vi "subcollect.vi"(2 "Firing Data":T1={"error"={"status"=FALSE, "code"=0, "source"=""}, "LeftWheelRefnum"={"DeviceStatus"={"status"=FALSE, "code"=0, "source"=""}, "Type"=enum."PWM", "PWM"={"PWM Channel"=enum."Invalid", "DeadBand"={"Name"="", "maxPositivePwm"=0, "minPositivePwm"=0, "centerPwm"=0, "maxNegativePwm"=0, "minNegativePwm"=0, "angularRange"=0}}, "CAN"={"Device Number"=0, "Control Mode"=enum."Percent VBus", "Semaphore"=refnum, "Max Vout"=12.0, "TalonSRX Control Mode"=enum."Percent VBus"}, "Invert"=FALSE}, "RightWheelRefnum"={"DeviceStatus"={"status"=FALSE, "code"=0, "source"=""}, "Type"=enum."PWM", "PWM"={"PWM Channel"=enum."Invalid", "DeadBand"={"Name"="", "maxPositivePwm"=0, "minPositivePwm"=0, "centerPwm"=0, "maxNegativePwm"=0, "minNegativePwm"=0, "angularRange"=0}}, "CAN"={"Device Number"=0, "Control Mode"=enum."Percent VBus", "Semaphore"=refnum, "Max Vout"=12.0, "TalonSRX Control Mode"=enum."Percent VBus"}, "Invert"=FALSE}, "PushSolenoidRefnum"={"DevStatus"={"status"=FALSE, "code"=0, "source"=""}, "Pneumatics Control Module"=0, "Forward Solenoid Channel"=enum."Invalid", "Reverse Solenoid Channel"=enum."Invalid"}, "AngleMotorPosition(t)"=0.0, "LaunchSpeed(t/100ms)"=0.0, "CollectSpeed(t/100ms)"=0.0, "SpinupDuration(10ms)"=0, "ShotDuration(10ms)"=0, "PowerScale"=0.0, "AngleShift"=0, "VisionPrepAngle"=0.0}, 3 "Manual Control":T11, 4 "CollectionTrigger":bool, 5 "SpinupTrigger":bool) -> (0 "Speed":dbl, 1 "Angle":dbl)   [LabVIEW 2015]
uses:
  Bundle.ctl
  <vilib>/Rock Robotics/WPI/MotorControl/WPI_MotorControlDeviceRef.ctl
  <vilib>/Rock Robotics/WPI/MotorControl/WPI_MotorControlType.ctl
  <vilib>/Rock Robotics/SystemInterfaces/DIO/FPGA_DIOPWMChannel.ctl
  <vilib>/Rock Robotics/WPI/PWM/WPI_PWMDeadband.ctl
  <vilib>/Rock Robotics/WPI/CAN/Jaguar/SubVIs/WPI_CANJaguar_ControlMode.ctl
  <vilib>/Rock Robotics/WPI/CAN/TalonSRX/WPI_CANTalonSRX_APIControlMode.ctl
  <vilib>/Rock Robotics/WPI/Solenoid/WPI_SolenoidDevRef.ctl
  <vilib>/Rock Robotics/WPI/Solenoid/WPI_SolenoidChannel.ctl
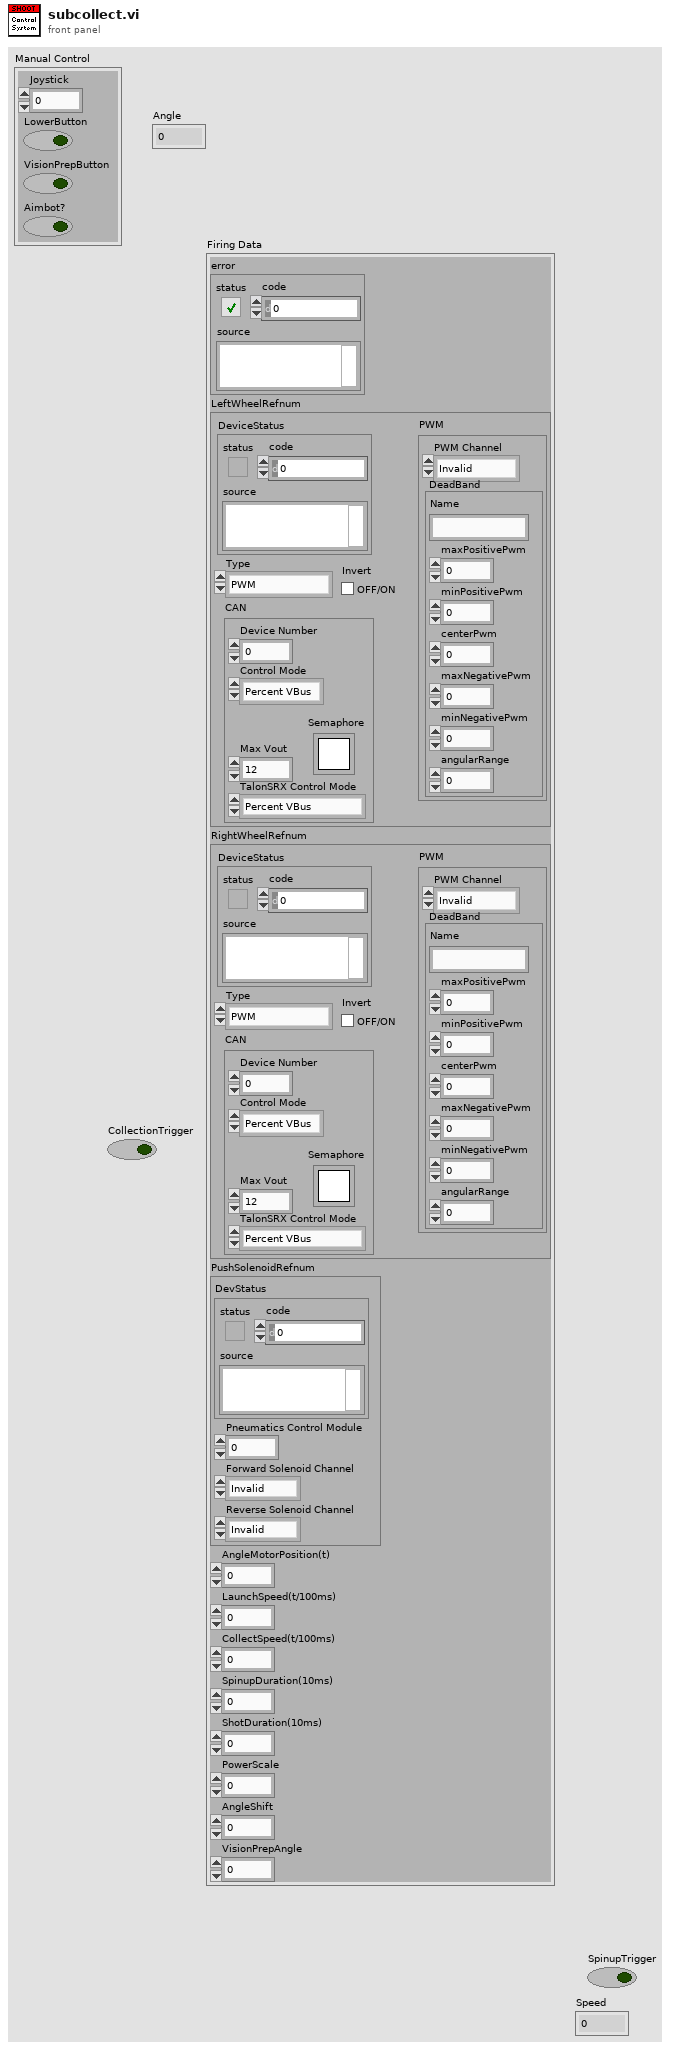
[diagram p1: front panel]
types:
  T1 = typedef "Bundle.ctl" = cluster{"error":errorcluster, "LeftWheelRefnum":T2, "RightWheelRefnum":T2, "PushSolenoidRefnum":T9, "AngleMotorPosition(t)":dbl, "LaunchSpeed(t/100ms)":dbl, "CollectSpeed(t/100ms)":dbl, "SpinupDuration(10ms)":i32, "ShotDuration(10ms)":i32, "PowerScale":dbl, "AngleShift":i32, "VisionPrepAngle":dbl}
  T2 = typedef "WPI_MotorControlDeviceRef.ctl" = cluster{"DeviceStatus":errorcluster, "Type":T3, "PWM":cluster{"PWM Channel":T4, "DeadBand":T5}, "CAN":cluster{"Device Number":u8, "Control Mode":T6, "Semaphore":T7, "Max Vout":dbl, "TalonSRX Control Mode":T8}, "Invert":bool}
  T3 = typedef "WPI_MotorControlType.ctl" = enum16{"PWM", "CAN", "CANTalonSRX"}
  T4 = typedef "FPGA_DIOPWMChannel.ctl" = enum8{"PWM 0", "PWM 1", "PWM 2", "PWM 3", "PWM 4", "PWM 5", "PWM 6", "PWM 7", "PWM 8", "PWM 9", "PWM MXP 0", "PWM MXP 1", "PWM MXP 2", "PWM MXP 3", "PWM MXP 4", "PWM MXP 5", "PWM MXP 6", "PWM MXP 7", "PWM MXP 8", "PWM MXP 9", "Invalid"}
  T5 = typedef "WPI_PWMDeadband.ctl" = cluster{"Name":string, "maxPositivePwm":i32, "minPositivePwm":i32, "centerPwm":i32, "maxNegativePwm":i32, "minNegativePwm":i32, "angularRange":u16}
  T6 = typedef "WPI_CANJaguar_ControlMode.ctl" = enum8{"Percent VBus", "Current", "Speed", "Position", "Voltage"}
  T7 = typedef "Semaphore RefNum" = refnum<k1>
  T8 = typedef "WPI_CANTalonSRX_APIControlMode.ctl" = enum8{"Percent VBus", "Speed", "Position", "Slave", "Unchanged / Invalid", "Voltage Compensation", "Current", "Motion Profile"}
  T9 = typedef "WPI_SolenoidDevRef.ctl" = cluster{"DevStatus":errorcluster, "Pneumatics Control Module":u8, "Forward Solenoid Channel":T10, "Reverse Solenoid Channel":T10}
  T10 = typedef "WPI_SolenoidChannel.ctl" = enum8{"Solenoid 0", "Solenoid 1", "Solenoid 2", "Solenoid 3", "Solenoid 4", "Solenoid 5", "Solenoid 6", "Solenoid 7", "Invalid"}
  T11 = cluster{"Joystick":dbl, "LowerButton":bool, "VisionPrepButton":bool, "Aimbot?":bool}
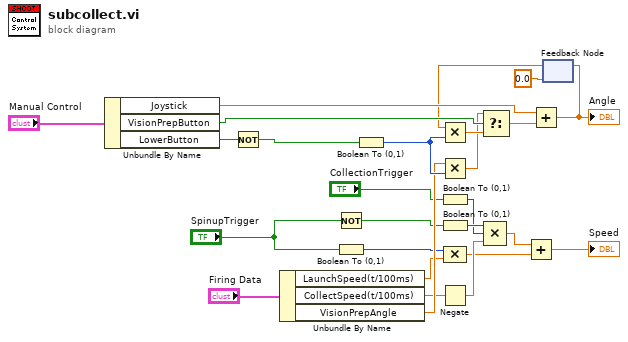
[diagram p0: block diagram]
diagram:
  n1 = Unbundle By Name("Manual Control") -> ("Joystick"=w19:dbl, "VisionPrepButton"=w26:bool, "LowerButton"=w25:bool)
  n2 = Not(x=w25) -> (.not. x?=w20:bool)
  n3 = Unbundle By Name("Firing Data") -> ("LaunchSpeed(t/100ms)"=w8:dbl, "CollectSpeed(t/100ms)"=w10:dbl, "VisionPrepAngle"=w16:dbl)
  n4 = Not(x="SpinupTrigger") -> (.not. x?=w11:bool)
  n5 = Boolean To (0,1)(Boolean="SpinupTrigger") -> (0, 1=w9:i16)
  n6 = Boolean To (0,1)(Boolean=w20) -> (0, 1=w22:i16)
  n7 = Multiply(x=w16, y=w22) -> (x*y=w21:dbl)
  n8 = Boolean To (0,1)(Boolean="CollectionTrigger") -> (0, 1=w14:i16)
  n9 = Boolean To (0,1)(Boolean=w11) -> (0, 1=w15:i16)
  n10 = Negate(x=w10) -> (-x=w13:dbl)
  n11 = Compound Arithmetic op=MULTIPLY(w9, w8) -> (w6:dbl)
  n12 = Compound Arithmetic op=MULTIPLY(w15, w14, w13) -> (w5:dbl)
  n13 = Add(x=w5, y=w6) -> (x+y=→"Speed":dbl)
  n14 = feedback #1(0.0 ("t")) -> (w3:dbl)
  n15 = Multiply(x=w3, y=w22) -> (x*y=w23:dbl)
  n16 = Select(t=w21, s=w26, f=w23) -> (s? t:f=w18:dbl)
  n17 = Add(x=w19, y=w18) -> (x+y=w1:dbl)
  "Angle" <- w1
  n18 = feedback-in #1(w1) -> ()
